vi "Update RX Slot Display.vi"(8 "error in":errorcluster, 9 "Location":cluster{"X":i32, "Y":i32}, 10 "Button":i32, 11 "UI Actor in":refnum<class "UI Actor.lvclass">) -> (0 "error out":errorcluster, 3 "UI Actor out":refnum<class "UI Actor.lvclass">)   [LabVIEW 2020, in "UI Actor.lvlib" / "UI Actor.lvclass"]
uses:
  UI Actor.lvclass
  UI Actor.lvclass/UI Actor.ctl
  PDO Grid/PDO Grid.lvclass
  D:/git/Sourcegrid-LabVIEW/source/Grid/SourceGrid.lvclass
  <vilib>/JDP Science/JSONtext/LVClass Serializer/JSONtext LVClass Serializer.lvclass
  Sourcegrid-LabVIEW/source/Cells/Cell/Cell.lvclass
  Sourcegrid-LabVIEW/source/Grid/SourceGrid.lvclass
  320aeeb9-ea85-43b7-8258-4ae750d7a996.vi
  Controls/RX Communication Parameter.ctl
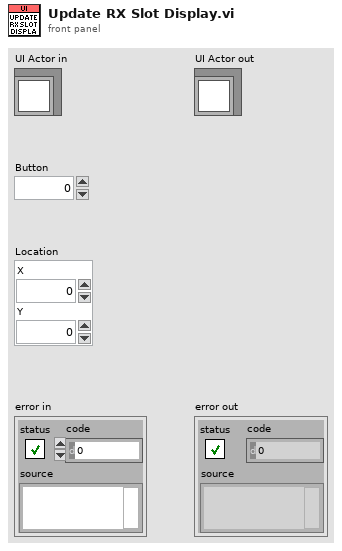
[diagram p1: front panel]
types:
  T1 = typedef "UI Actor.lvlib/UI Actor.lvclass/RX Communication Parameter.ctl" = cluster{"Communication":u16, "Mapping":u16, "COB":u32, "Transm. Type":u8, "Inhibit":u16, "Event Timer":u16, "Sync Start":u8}
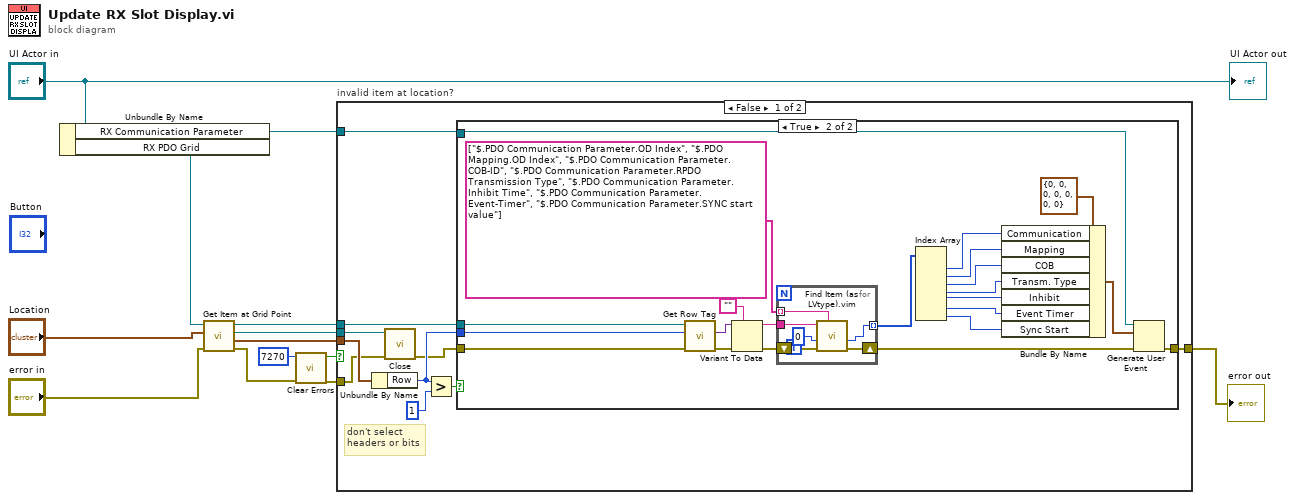
[diagram p0: block diagram]
diagram:
  n1 = Unbundle By Name("UI Actor in") -> ("RX Communication Parameter"=w5:refnum<user-event>, "RX PDO Grid"=w12:refnum<class "PDO Grid.lvclass">)
  n2 = call "Get Item at Grid Point.vi"("error in"="error in", "Location"="Location", "SourceGrid in"=w12) -> ("error out"=w3:errorcluster, "Cell Position"=w9:cluster{"Row":i32, "Column":i32}, "Cell out"=w6:refnum<class "Cell.lvclass">, "SourceGrid out"=w8:refnum<class "PDO Grid.lvclass">)  [unwired: 5 in]
  n3 = call <vilib>:"Clear Errors.vi"("error in (no error)"=w3, "specific error code to clear (0: all)"=7270) -> ("error out"=w2:errorcluster, "specific error cleared?"=w1:bool)  [unwired: 4 in]
  n4 = case "invalid item at location?" shown="False" w1 {
    tunnel: w9 -> [w23 _]
    tunnel: w8 -> [w21 _]
    tunnel: [w14 w53] -> w7
    tunnel: w6 -> [w18 _]
    tunnel: w5 -> [w17 _]
    tunnel: w2 -> [w16 w53]
    frame False {
      # "don't select\nheaders or bits"
      n5 = Unbundle By Name(w23) -> ("Row"=w20:i32)
      n6 = call-dynamic "Close.vi"("error in"=w16, "Cell in"=w18) -> ("error out"=w19:errorcluster)  [unwired: 8 in, 1 out]
      n7 = Greater?(x=w20, y=1) -> (0:w15:bool)
      n8 = case shown="True" w15 {
        tunnel: w21 -> [_ w46]
        tunnel: w20 -> [_ w44]
        tunnel: w19 -> [w24 w43]
        tunnel: w17 -> [_ w42]
        tunnel: [w24 w45] -> w14
        frame False {
        }
        frame True {
          n9 = call "Get Row Tag.vi"("error in"=w43, "Row Index"=w44, "SourceGrid in"=w46) -> ("error out"=w41:errorcluster, "object"=w40:variant)  [unwired: 6 in, 1 out]
          n10 = Variant To Data(error in=w41, type="", Variant=w40) -> (data=w38:string, error out=w36:errorcluster)
          n11 = for {
            tunnel: w38 -> [w49]
            tunnel: string[] ["$.PDO Communication Parameter.OD Index", "$.PDO Mapping.OD Index", "$.PDO Communication Parameter.COB-ID", "$.PDO Communication Parameter.RPDO Transmission Type", "$.PDO Communication Parameter.Inhibit Time", "$.PDO Communication Parameter.Event-Timer", "$.PDO Communication Parameter.SYNC start value"] -> [w52] mode=indexing
            shift-right: [w50] -> w35
            shift-left: w36 -> [w51]
            tunnel: [w48] -> w32 mode=indexing
            n12 = call "Find Item (as LVtype).vim"("$Path or Item Name"=w52, "error in (no error)"=w51, "Data Type and Default Value"=u32 0, "JSON"=w49) -> ("error out"=w50:errorcluster, "Data"=w48:u32)  [unwired: 4 in, 2 out]
          }
          n13 = Index Array(array=w32) -> (element #1=w31:u32, element #2=w30:u32, element #3=w29:u32, element #4=w28:u32, element #5=w27:u32, element #6=w26:u32, element #7=w25:u32)  [unwired: 7 in]
          n14 = Bundle By Name(cluster=T1 {"Communication"=0, "Mapping"=0, "COB"=0, "Transm. Type"=0, "Inhibit"=0, "Event Timer"=0, "Sync Start"=0} ("event data"), "Communication"=w31, "Mapping"=w30, "COB"=w29, "Transm. Type"=w28, "Inhibit"=w27, "Event Timer"=w26, "Sync Start"=w25) -> (w33:T1)
          n15 = Generate User Event(user event=w42, event data cluster=w33, error in=w35) -> (error out=w45:errorcluster)  [unwired: 1 in, 1 out]
        }
      }
    }
    frame True {
      # "No Cell at given location"
    }
  }
  "error out" <- w7
  "UI Actor out" <- "UI Actor in"
